vi "Read from device.vi"() -> (2 "Humidity":dbl, 3 "temperature":dbl)   [LabVIEW 2016]
uses:
  RDingUSB.dll
panel:
  out "error out":errorcluster
  in  "Specify location":string
  in  "stop":bool
  out "Read work?":bool
  out "Write work?":bool
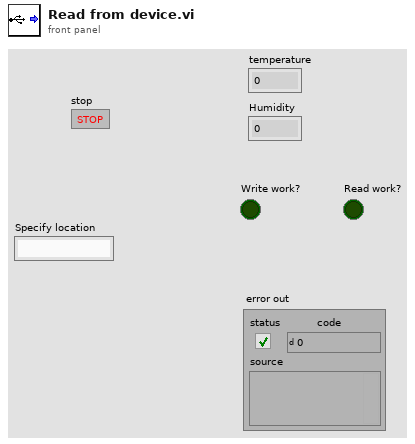
[diagram p1: front panel]
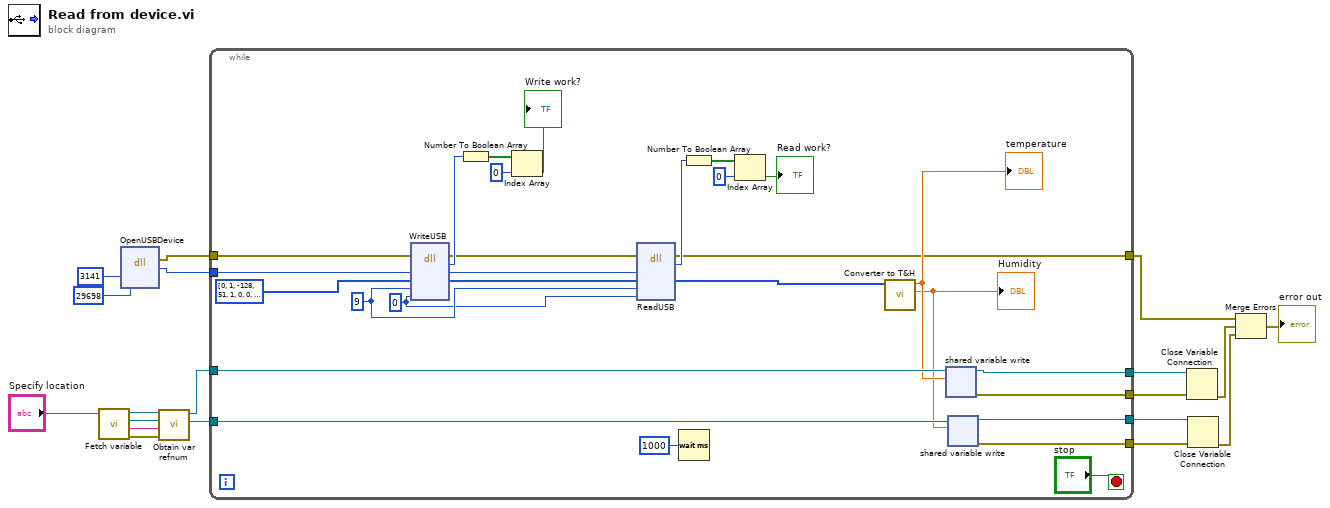
[diagram p0: block diagram]
diagram:
  n1 = call "Fetch variable.vi"("Specify location"="Specify location") -> ("error out"=w15:errorcluster, "machine name"=w12:string, "Humidity var"=w13:refnum<k21>, "Temperature var"=w14:refnum<k21>)  [unwired: 7 in]
  n2 = dll-call lib="C:/Users/Voodoo/Desktop/Shan.hao/TEMPerHUM via DLL/RDingUSB.dll" fn="OpenUSBDevice"("VID"=3141, "PID"=29698) -> (error out=w5:errorcluster, "return type"=w17:i64)  [unwired: 5 in, 1 out]
  n3 = call "Obtain var refnum.vi"("error in (no error)"=w15, "machine name"=w12, "Humidity var"=w13, "Temperature var"=w14) -> ("Humidity Refnum"=w10:refnum<k21>, "Temperature Refnum"=w11:refnum<k21>)  [unwired: 5 in, 1 out]
  n4 = while {
    tunnel: w17 -> [w31]
    tunnel: w11 -> [w30]
    tunnel: w10 -> [w29]
    tunnel: [w26] -> w9
    tunnel: [w25] -> w8
    tunnel: [w24] -> w7
    tunnel: [w23] -> w6
    tunnel: w5 -> [w22]
    tunnel: [w20] -> w4
    stop <- "stop" stop-if-true
    w32 = u64 0 ("number0fBytesWrite")
    w34 = 9 ("bytesCount")
    n5 = dll-call lib="C:/Users/Voodoo/Desktop/Shan.hao/TEMPerHUM via DLL/RDingUSB.dll" fn="WriteUSB"(error in=w22, "deviceHandle"=w31, "buffer"=i8[] [0, 1, -128, 51, 1, 0, 0, 0, 0] ("Array"), "bytesCount"=w34, "number0fBytesWrite"=w32) -> (error out=w21:errorcluster, "return type"=w37:i32, "deviceHandle"=w35:i64, "buffer"=w33:i8[])  [unwired: 4 in, 1 out]
    n6 = Number To Boolean Array(number=w37) -> (Boolean array=w38:bool[])
    n7 = Index Array(array=w38, index=0) -> (element=→"Write work?":bool)
    n8 = dll-call lib="C:/Users/Voodoo/Desktop/Shan.hao/TEMPerHUM via DLL/RDingUSB.dll" fn="ReadUSB"(error in=w21, "deviceHandle"=w35, "buffer"=w33, "bytesCount"=w34, "number0fBytesRead"=w32) -> (error out=w20:errorcluster, "return type"=w44:i32, "buffer"=w45:u8[])  [unwired: 5 in, 1 out]
    n9 = Wait (ms)(milliseconds to wait=u32 1000) -> ()  [unwired: 1 out]
    n10 = Number To Boolean Array(number=w44) -> (Boolean array=w43:bool[])
    n11 = Index Array(array=w43, index=0) -> (element=→"Read work?":bool)
    n12 = call "Converter to T&H.vi"("buffer"=w45) -> ("Numeric"=w27:dbl, "Numeric 2"=w28:dbl)  [unwired: 9 in]
    "temperature" <- w28
    "Humidity" <- w27
    n13 = shared-variable-write(w30, w28) -> (w26:refnum<k21>, w23:errorcluster)  [unwired: 1 in]
    n14 = shared-variable-write(w29, w27) -> (w25:refnum<k21>, w24:errorcluster)  [unwired: 1 in]
  }
  n15 = Close Variable Connection(8:w6, 11:w9) -> (0:w3:errorcluster)
  n16 = Close Variable Connection(8:w7, 11:w8) -> (0:w2:errorcluster)
  n17 = Merge Errors(w4, w3, w2) -> (→"error out":errorcluster)
